vi "Remove points in historam by half width.vi"() -> ()   [LabVIEW 2021]
uses:
  <vilib>/Utility/file.llb/Read Delimited Spreadsheet (DBL).vi
  <vilib>/Utility/file.llb/Write Delimited Spreadsheet (DBL).vi
  <vilib>/Analysis/NI_AALPro.lvlib
  <vilib>/gmath/NI_Gmath.lvlib
panel:
  in  "Refuse value":dbl format="%#_13g"
  in  "# bins":i32=100
  in  "File name suffix":string(combo)="_reduced"
  in  "Number of Half width":dbl=3.0 format="%#_13g"
  out "Progress %":dbl=98.36065573770492
  in  "book number":i32=475
  in  "file path (dialog if empty)":path=path "C:/Users/gyue/Box/Guang Yue uiuc research box folder/data/Contour plot"
  # "Remove data points smaller than Peak-half width"
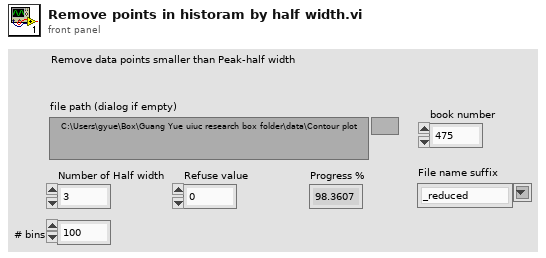
[diagram p1: front panel]
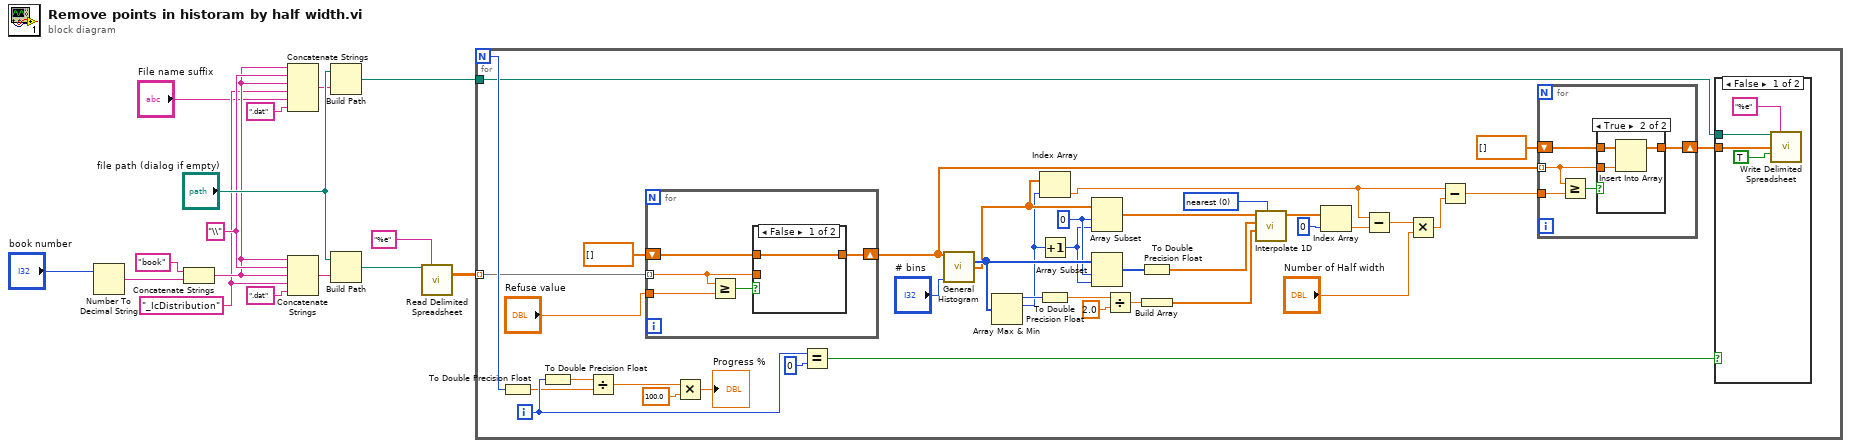
[diagram p0: block diagram]
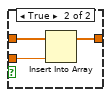
[diagram p2: hidden frame]
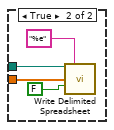
[diagram p3: hidden frame]
diagram:
  w5 = "_IcDistribution" ("string")
  w7 = "\\" ("string")
  n1 = Number To Decimal String(number="book number") -> (decimal integer string=w14:string)  [unwired: 1 in]
  n2 = Concatenate Strings("book" ("string"), w14) -> (w6:string)
  n3 = Concatenate Strings(w6, w7, w6, w5, "File name suffix", ".dat" ("string")) -> (w4:string)
  n4 = Concatenate Strings(w6, w7, w6, w5, ".dat" ("string")) -> (w15:string)
  n5 = Build Path(base path="file path (dialog if empty)", name or relative path=w4) -> (appended path=w3:path)
  n6 = Build Path(base path="file path (dialog if empty)", name or relative path=w15) -> (appended path=w16:path)
  n7 = call-poly <vilib>:"Read Delimited Spreadsheet.vi"("file path (dialog if empty)"=w16, "format (%.3f)"="%e") -> ("all rows"=w10:dbl[][])  [unwired: 8 in, 5 out]
  n8 = for {
    N -> [w55]
    tunnel: w10 -> [w19] mode=indexing
    tunnel: w3 -> [w45]
    i -> [w50]
    w38 = 0 items=["nearest", "linear", "spline", "cubic Hermite", "Lagrange"] ("method")
    w35 = 0 ("index")
    n9 = To Double Precision Float(number=w55) -> (double precision float=w46:dbl)
    n10 = To Double Precision Float(number=w50) -> (double precision float=w47:dbl)
    n11 = Divide(x=w47, y=w46) -> (x/y=w54:dbl)
    n12 = for {
      tunnel: w19 -> [w58] mode=indexing
      shift-right: [w59] -> w17
      shift-left: dbl[] [] -> [w60]
      tunnel: "Refuse value" -> [w57]
      n13 = Greater Or Equal?(x=w58, y=w57) -> (x >= y?=w56:bool)
      n14 = case shown="False" w56 {
        tunnel: w58 -> [_ w63]
        tunnel: w60 -> [w61 w64]
        tunnel: [w61 w62] -> w59
        frame False {
        }
        frame True {
          n15 = Insert Into Array(array=w64, new element=w63) -> (w62:dbl[])  [unwired: 1 in]
        }
      }
    }
    n16 = Multiply(x=w54, y=100.0) -> (x*y=→"Progress %":dbl)
    n17 = Equal?(x=w50, y=0) -> (x = y?=w48:bool)
    n18 = call <vilib>:"General Histogram.vi"("X"=w17, "# bins"="# bins") -> ("Histogram"=w39:i32[], "Axis"=w30:dbl[])  [unwired: 9 in, 3 out]
    n19 = Array Max & Min(array=w39) -> (max value=w42:i32, max index (indices)=w29:i32)  [unwired: 2 out]
    n20 = Index Array(array=w30, index=w29) -> (element=w23:dbl)
    n21 = Increment(x=w29) -> (x+1=w34:i32)
    n22 = To Double Precision Float(number=w42) -> (double precision float=w40:dbl)
    n23 = Array Subset(array=w30, index=w35, length=w34) -> (w33:dbl[])
    n24 = Array Subset(array=w39, index=w35, length=w34) -> (w37:i32[])
    n25 = Divide(x=w40, y=2.0) -> (x/y=w32:dbl)
    n26 = To Double Precision Float(number=w37) -> (double precision float=w36:dbl[])
    n27 = Build Array(w32) -> (w31:dbl[])
    n28 = call <vilib>:"Interpolate 1D.vi"("method"=w38, "xi"=w31, "X"=w36, "Y"=w33) -> ("yi"=w28:dbl[])  [unwired: 5 in, 2 out]
    n29 = Index Array(array=w28, index=0) -> (element=w27:dbl)
    n30 = Subtract(x=w23, y=w27) -> (x-y=w25:dbl)
    n31 = Multiply(x=w25, y="Number of Half width") -> (x*y=w22:dbl)
    n32 = Subtract(x=w23, y=w22) -> (x-y=w21:dbl)
    n33 = for {
      tunnel: w17 -> [w75] mode=indexing
      shift-right: [w76] -> w44
      shift-left: dbl[] [] -> [w77]
      tunnel: w21 -> [w74]
      n34 = Greater Or Equal?(x=w75, y=w74) -> (x >= y?=w73:bool)
      n35 = case shown="True" w73 {
        tunnel: w75 -> [_ w80]
        tunnel: w77 -> [w78 w81]
        tunnel: [w78 w79] -> w76
        frame False {
        }
        frame True {
          n36 = Insert Into Array(array=w81, new element=w80) -> (w79:dbl[])  [unwired: 1 in]
        }
      }
    }
    n37 = case shown="False" w48 {
      tunnel: w45 -> [w65 w72]
      tunnel: w44 -> [w66 w69]
      frame False {
        n38 = call-poly <vilib>:"Write Delimited Spreadsheet.vi"("file path (dialog if empty)"=w65, "format (%.3f)"="%e" ("format (%d)"), "1D data"=w66, "append to file? (new file:F)"=TRUE) -> ()  [unwired: 10 in, 2 out]
      }
      frame True {
        n39 = call-poly <vilib>:"Write Delimited Spreadsheet.vi"("file path (dialog if empty)"=w72, "format (%.3f)"="%e" ("format (%d)"), "1D data"=w69, "append to file? (new file:F)"=FALSE) -> ()  [unwired: 10 in, 2 out]
      }
    }
  }
